vi "Send.vi"(0 "STOMP in":refnum<class "STOMP.lvclass">, 1 "Destination":string, 2 "Body":string, 3 "headers":T1[](array[typedef]), 5 "error in (no error)":errorcluster, 6 "Receipt?":bool) -> (14 "STOMP out":refnum<class "STOMP.lvclass">, 19 "error out":errorcluster)   [LabVIEW 2017, in "LabVIEW STOMP.lvlib" / "STOMP.lvclass"]
uses:
  STOMP.lvclass
  Typedefs/Type_FrameHeader.ctl
  Typedefs/Type_ClientFrame.ctl
  Typedefs/Type_ClientFrameType.ctl
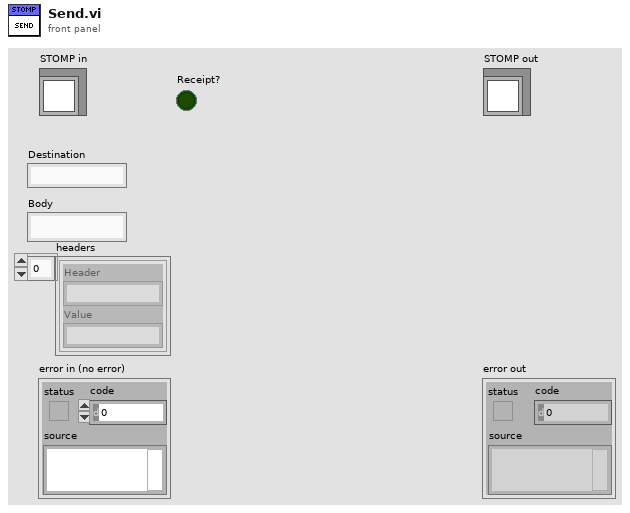
[diagram p1: front panel]
types:
  T1 = typedef "LabVIEW STOMP.lvlib/STOMP.lvclass/Type_FrameHeader.ctl" = cluster{"Header":string, "Value":string}
  T2 = typedef "LabVIEW STOMP.lvlib/STOMP.lvclass/Type_ClientFrameType.ctl" = enum16{"Undefined", "SEND", "SUBSCRIBE", "UNSUBSCRIBE", "BEGIN", "COMMIT", "ABORT", "ACK", "NACK", "DISCONNECT"}
  T3 = typedef "LabVIEW STOMP.lvlib/STOMP.lvclass/Type_ClientFrame.ctl" = cluster{"Type":T2, "Headers":T1[], "Body":string}
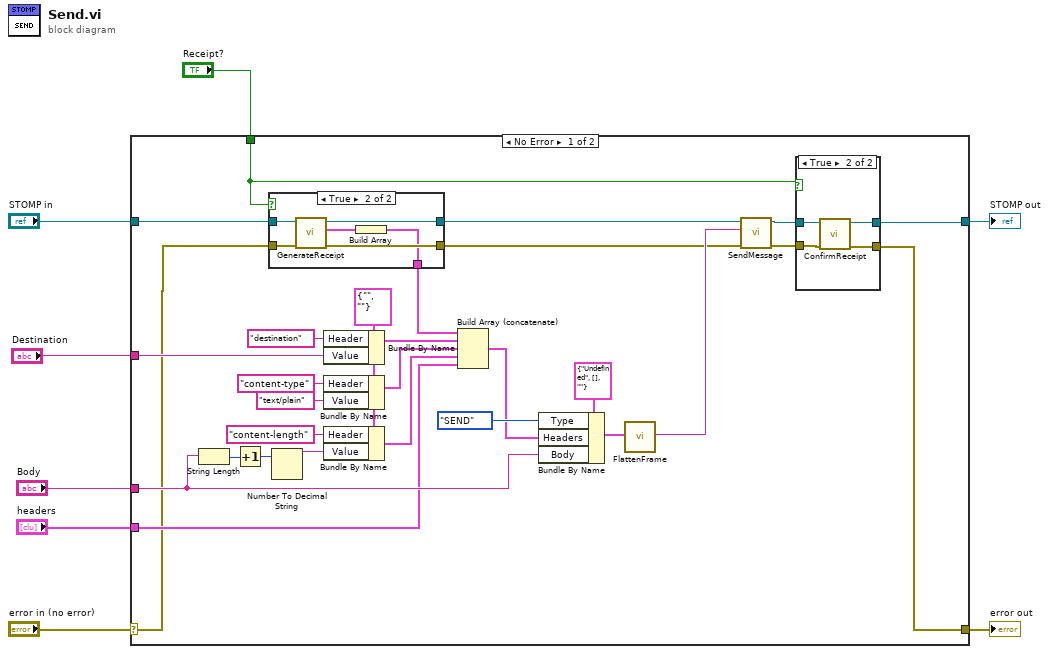
[diagram p0: block diagram]
diagram:
  n1 = case shown="No Error" "error in (no error)" {
    selector: "error in (no error)" -> [w17 w53]
    tunnel: [w11 w53] -> w7
    tunnel: [w10 w52] -> w5
    tunnel: "STOMP in" -> [w18 w52]
    tunnel: "Destination" -> [w35 _]
    tunnel: "Body" -> [w27 _]
    tunnel: "headers" -> [w20 _]
    tunnel: "Receipt?" -> [w9 _]
    frame No Error {
      w19 = T1 {"Header"="", "Value"=""}
      n2 = String Length(string=w27) -> (length=w26:i32)
      n3 = Increment(x=w26) -> (x+1=w21:i32)
      n4 = case shown="True" w9 {
        tunnel: w18 -> [w45 w51]
        tunnel: w17 -> [w44 w50]
        tunnel: [w45 w49] -> w16
        tunnel: [w44 w48] -> w15
        tunnel: [_ w46] -> w14
        frame False {
        }
        frame True {
          n5 = call-dynamic "GenerateReceipt.vi"("error in (no error)"=w50, "STOMP in"=w51) -> ("error out"=w48:errorcluster, "Receipt Header"=w47:T1, "STOMP out"=w49:refnum<class "STOMP.lvclass">)  [unwired: 7 in]
          n6 = Build Array(w47) -> (w46:T1[])
        }
      }
      n7 = Number To Decimal String(number=w21) -> (decimal integer string=w25:string)  [unwired: 1 in]
      n8 = Bundle By Name(cluster=w19, "Header"="destination", "Value"=w35) -> (w31:T1)
      n9 = Bundle By Name(cluster=w19, "Header"="content-type", "Value"="text/plain") -> (w30:T1)
      n10 = Bundle By Name(cluster=w19, "Header"="content-length", "Value"=w25) -> (w22:T1)
      n11 = Build Array (concatenate)(w14, w31, w30, w22, w20) -> (w29:T1[])
      n12 = Bundle By Name(cluster=T3 {"Type"=enum."Undefined", "Headers"=[], "Body"=""} ("Type_ClientFrame"), "Type"=Type_ClientFrameType."SEND", "Headers"=w29, "Body"=w27) -> (w24:T3)
      n13 = call "FlattenFrame.vi"("Client Frame"=w24) -> ("flattened frame"=w23:string)  [unwired: 18 in]
      n14 = call-dynamic "SendMessage.vi"("error in (no error)"=w15, "data in"=w23, "STOMP in"=w16) -> ("error out"=w12:errorcluster, "STOMP out"=w13:refnum<class "STOMP.lvclass">)  [unwired: 7 in]
      n15 = case shown="True" w9 {
        tunnel: w13 -> [w38 w43]
        tunnel: w12 -> [w39 w42]
        tunnel: [w39 w41] -> w11
        tunnel: [w38 w40] -> w10
        frame False {
        }
        frame True {
          n16 = call-dynamic "ConfirmReceipt.vi"("error in (no error)"=w42, "STOMP in"=w43) -> ("error out"=w41:errorcluster, "STOMP out"=w40:refnum<class "STOMP.lvclass">)  [unwired: 8 in]
        }
      }
    }
    frame Error {
    }
  }
  "error out" <- w7
  "STOMP out" <- w5
